vi "ReadNet_Automatic.vi"(8 "error in":errorcluster, 9 "framework":string, 10 "ConfigPath":path, 11 "ModelPath":path) -> (0 "error out":errorcluster, 3 "NET":refnum<class "NET.lvclass">)   [LabVIEW 2020, in "OpenLvVision_OpenCv.lvlib"]
doc: "Read deep learning network represented in one of the supported formats."
uses:
  OpenLvVision_OpenCv.lvlib
  NET/NET.lvclass
  _LvHelpers/EdvrObject/TypeDef/Edvr.ctl
  _LvHelpers/EdvrObject/EdvrObject.lvclass
  Dlls/OlvOpenCvWrapper.dll
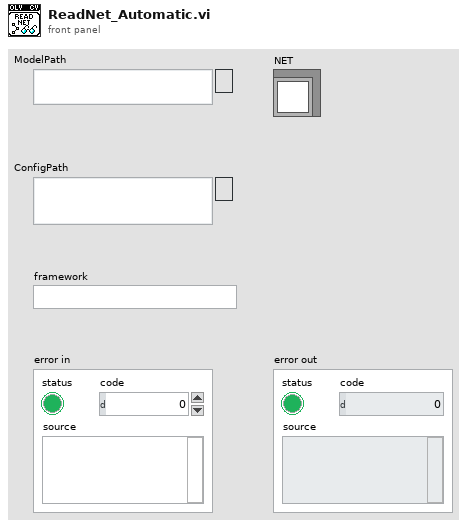
[diagram p1: front panel]
types:
  T1 = typedef "OpenLvVision_OpenCv.lvlib/EdvrObject.lvclass/Edvr.ctl" = refnum<data-value>
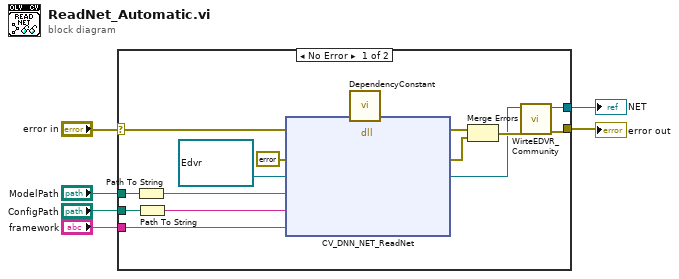
[diagram p0: block diagram]
diagram:
  n1 = case shown="No Error" "error in" {
    selector: "error in" -> [w16 w21]
    tunnel: [w14 w21] -> w5
    tunnel: [w12 _] -> w4
    tunnel: "ModelPath" -> [w10 _]
    tunnel: "ConfigPath" -> [w8 _]
    tunnel: "framework" -> [w11 _]
    frame No Error {
      n2 = Path To String(path=w10) -> (string=w9:string)
      n3 = Path To String(path=w8) -> (string=w7:string)
      n4 = dll-call lib="C:/Users/lukas/Downloads/OpenLvVision_OpenCv/SourceCode/LabView/OpenLvVision_OpenCv/Dlls/OlvOpenCvWrapper.dll" fn="CV_DNN_NET_ReadNet"(error in=w16, "Error"=errorcluster {"status"=FALSE, "code"=0, "source"=""} ("error out"), "edvrRef"=T1 refnum ("Edvr"), "modelPath"=w9, "configPath"=w7, "framework"=w11) -> (error out=w19:errorcluster, "Error"=w18:errorcluster, "edvrRef"=w13:T1)  [unwired: 6 in, 1 out]
      n5 = call "DependencyConstant.vi"() -> ()  [unwired: 12 in]
      n6 = Merge Errors(w19, w18) -> (w15:errorcluster)
      n7 = call "WirteEDVR_Community.vi"("error in"=w15, "Edvr"=w13) -> ("error out"=w14:errorcluster, "NET"=w12:refnum<class "NET.lvclass">)  [unwired: 8 in]
    }
    frame Error {
    }
  }
  "NET" <- w4
  "error out" <- w5
